vi "ListTables.vi"(8 "error in (no error)":errorcluster, 11 "DbPath":path) -> (0 "error out":errorcluster, 1 "OK？":bool, 2 "Tables":string[](array[string]), 3 "DbPathout":path)   [LabVIEW 2017]
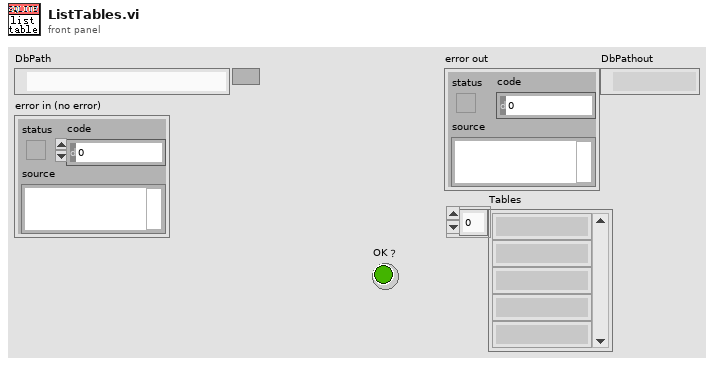
[diagram p1: front panel]
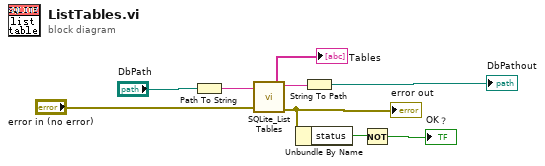
[diagram p0: block diagram]
diagram:
  n1 = Path To String(path="DbPath") -> (string=w9:string)
  n2 = call "SQLite_List Tables.vi"("DB Path"=w9, "error in (no error)"="error in (no error)") -> ("Tables"=→"Tables":string[], "DB Path Out"=w6:string, "error out"=w3:errorcluster)  [unwired: 6 in]
  "error out" <- w3
  n3 = Unbundle By Name(w3) -> ("status"=w2:bool)
  n4 = String To Path(string=w6) -> (path=→"DbPathout":path)
  n5 = Not(x=w2) -> (.not. x?=→"OK？":bool)
